vi "FTDI_MPSSE_Close.vi"(8 "error in (no error)":errorcluster, 11 "Handler":u32) -> (0 "error out":errorcluster)   [LabVIEW 2018]
uses:
  dll/libMPSSE.dll
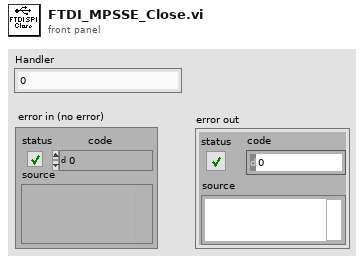
[diagram p1: front panel]
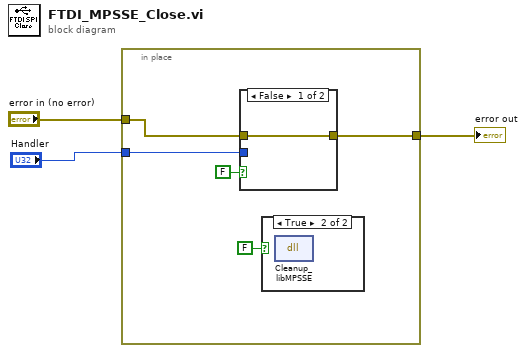
[diagram p0: block diagram]
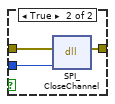
[diagram p2: hidden frame]
diagram:
  n1 = in-place {
    in-place-border: "error in (no error)" -> [w8]
    in-place-border: [w7] -> w2
    in-place-border: "Handler" -> [w6]
    n2 = case shown="False" FALSE {
      tunnel: w8 -> [w9 w12]
      tunnel: [w9 w11] -> w7
      tunnel: w6 -> [_ w10]
      frame False {
      }
      frame True {
        n3 = dll-call lib="D:/LABVIEW/SEQUENSER_SNA/Ver_12/FTDI SPI/dll/libMPSSE.dll" fn="SPI_CloseChannel"(error in=w12, "handle"=w10) -> (error out=w11:errorcluster)  [unwired: 4 in, 1 out]
      }
    }
    n4 = case shown="True" FALSE {
      frame False {
      }
      frame True {
        n5 = dll-call lib="D:/LABVIEW/SEQUENSER_SNA/Ver_12/FTDI SPI/dll/libMPSSE.dll" fn="Cleanup_libMPSSE"() -> ()  [unwired: 4 in, 2 out]
      }
    }
  }
  "error out" <- w2
